vi "Digital Pattern Gen 1.3 In Place Input Write Structure.vi"(5 "Device Inputs":dbl[](array[numeric]), 7 "Last Device Inputs":dbl[](array[numeric]), 8 "error in (no error)":errorcluster, 9 "FPGA ref in":T1, 11 "1.3 Digital Pattern Gen in":T2) -> (0 "error out":errorcluster, 1 "FPGA ref out":T1, 3 "1.3 Digital Pattern Gen out":T2)   [LabVIEW 2013, in "Engine Simulation Toolkit Engine.lvlib"]
uses:
  Engine Simulation Toolkit Engine.lvlib
  Shared/1.3 Digital Pattern Gen Engine Data.ctl
  Shared/1.3 Digital Pattern Gen FIFO Idxs.ctl
  Digital Pattern Gen 1.0 Input Ref.ctl
  Digital Pattern Gen 1.0 FPGA Inputs Write Node.vi
  Shared/Engine Simulation Toolkit Shared.lvlib
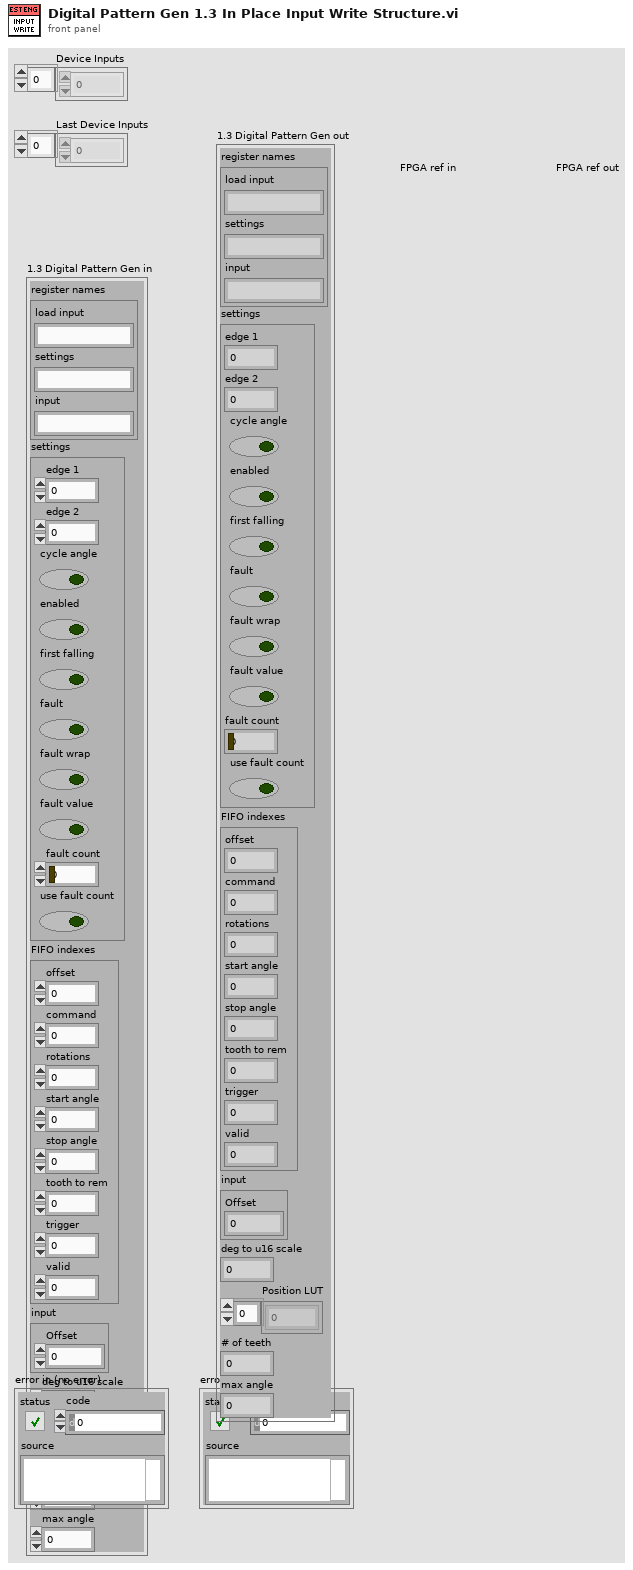
[diagram p1: front panel]
types:
  T1 = typedef "Engine Simulation Toolkit Engine.lvlib/Digital Pattern Gen 1.0 Input Ref.ctl" = refnum<k20>
  T2 = typedef "Engine Simulation Toolkit Shared.lvlib/1.3 Digital Pattern Gen Engine Data.ctl" = cluster{"register names":cluster{"load input":string, "settings":string, "input":string}, "settings":cluster{"edge 1":u16, "edge 2":u16, "cycle angle":bool, "enabled":bool, "first falling":bool, "fault":bool, "fault wrap":bool, "fault value":bool, "fault count":fxp<+,4,4>, "use fault count":bool}, "FIFO indexes":T3, "input":cluster{"Offset":i16}, "deg to u16 scale":dbl, "Position LUT":u16[], "# of teeth":i16, "max angle":dbl}
  T3 = typedef "Engine Simulation Toolkit Shared.lvlib/1.3 Digital Pattern Gen FIFO Idxs.ctl" = cluster{"offset":i32, "command":i32, "rotations":i32, "start angle":i32, "stop angle":i32, "tooth to rem":i32, "trigger":i32, "valid":i32}
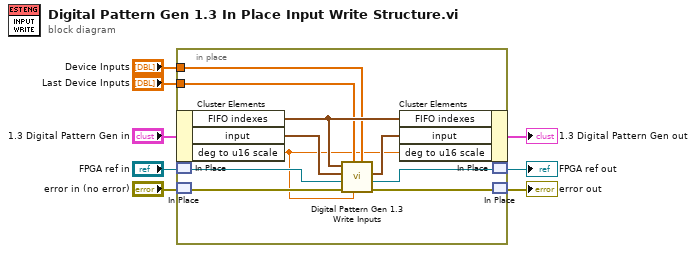
[diagram p0: block diagram]
diagram:
  n1 = in-place {
    in-place-border: "Last Device Inputs" -> [w13]
    in-place-border: "Device Inputs" -> [w12]
    n2 = in-place-cluster #1("1.3 Digital Pattern Gen in") -> ("FIFO indexes"=w15:T3, "input"=w16:cluster{"Offset":i16}, "deg to u16 scale"=w9:dbl)
    n3 = in-place-match #2("FPGA ref in") -> (w11:T1)
    n4 = in-place-match #3("error in (no error)") -> (w18:errorcluster)
    n5 = call "Digital Pattern Gen 1.3 Write Inputs.vi"("Device inputs"=w12, "offset convert"=w9, "Last Device inputs"=w13, "error in (no error)"=w18, "input reference in"=w11, "input in"=w16, "FIFO indexes.inputs"=w15) -> ("error out"=w17:errorcluster, "input reference out"=w10:T1, "input out"=w14:cluster{"Offset":i16})  [unwired: 2 in]
    n6 = in-place-cluster #1("FIFO indexes"=w15, "input"=w14, "deg to u16 scale"=w9) -> (→"1.3 Digital Pattern Gen out":T2)
    n7 = in-place-match #2(w10) -> (→"FPGA ref out":T1)
    n8 = in-place-match #3(w17) -> (→"error out":errorcluster)
  }
